vi "Finish.vi"   [LabVIEW 2015]
doc: "This VI is called just before exiting. It is expected to close I/O refnum, save collected data, etc."
uses:
  Device Refnums.ctl
  <vilib>/Rock Robotics/WPI/Utilities/WPI_GetSetVariantRefNum.vi
  ADIS16448-RoboRIO-Driver/trunk/LabVIEW/ADI MXP IMU/FRC ADI MXP IMU.lvlib
types:
  T1 = typedef "Device Refnums.ctl" = string
  T2 = typedef "WPI_JoystickDevRef.ctl" = cluster{"Device":T3}
  T3 = typedef "WPI_JoystickDeviceEnum.ctl" = enum16{"USB 0", "USB 1", "USB 2", "USB 3", "USB 4", "USB 5"}
  T4 = typedef "WPI_RobotDriveDevRef.ctl" = cluster{"DevStatus":errorcluster, "Motors[]":T5[], "Square Inputs":bool, "Max Output":dbl}
  T5 = typedef "WPI_MotorControlDeviceRef.ctl" = cluster{"DeviceStatus":errorcluster, "Type":T6, "PWM":cluster{"PWM Channel":T7, "DeadBand":T8}, "CAN":cluster{"Device Number":u8, "Control Mode":T9, "Semaphore":T10, "Max Vout":dbl, "TalonSRX Control Mode":T11}, "Invert":bool}
  T6 = typedef "WPI_MotorControlType.ctl" = enum16{"PWM", "CAN", "CANTalonSRX"}
  T7 = typedef "FPGA_DIOPWMChannel.ctl" = enum8{"PWM 0", "PWM 1", "PWM 2", "PWM 3", "PWM 4", "PWM 5", "PWM 6", "PWM 7", "PWM 8", "PWM 9", "PWM MXP 0", "PWM MXP 1", "PWM MXP 2", "PWM MXP 3", "PWM MXP 4", "PWM MXP 5", "PWM MXP 6", "PWM MXP 7", "PWM MXP 8", "PWM MXP 9", "Invalid"}
  T8 = typedef "WPI_PWMDeadband.ctl" = cluster{"Name":string, "maxPositivePwm":i32, "minPositivePwm":i32, "centerPwm":i32, "maxNegativePwm":i32, "minNegativePwm":i32, "angularRange":u16}
  T9 = typedef "WPI_CANJaguar_ControlMode.ctl" = enum8{"Percent VBus", "Current", "Speed", "Position", "Voltage"}
  T10 = typedef "Semaphore RefNum" = refnum<k1>
  T11 = typedef "WPI_CANTalonSRX_APIControlMode.ctl" = enum8{"Percent VBus", "Speed", "Position", "Slave", "Unchanged / Invalid", "Voltage Compensation", "Current", "Motion Profile"}
  T12 = typedef "WPI_EncoderDevRef.ctl" = cluster{"DevStatus":errorcluster, "EncoderIndex":T13, "CounterIndex":T14, "DistancePerCount":dbl, "Decoding Type":T15}
  T13 = typedef "FPGA_EncoderIdx.ctl" = enum8{"Enc 0", "Enc 1", "Enc 2", "Enc 3", "Enc 4", "Enc 5", "Enc 6", "Enc 7", "Invalid"}
  T14 = typedef "FPGA_CounterCtrSystemIndex.ctl" = enum8{"Ctr 0", "Ctr 1", "Ctr 2", "Ctr 3", "Ctr 4", "Ctr 5", "Ctr 6", "Ctr 7", "Invalid"}
  T15 = typedef "WPI_EncoderType.ctl" = enum16{"1x", "2x", "4x"}
  T16 = typedef "WPI_AnalogChannelDevRef.ctl" = cluster{"DevStatus":errorcluster, "Analog Channel":T17}
  T17 = typedef "FPGA_AIChannel.ctl" = enum8{"AI 0", "AI 1", "AI 2", "AI 3", "AI MXP 0", "AI MXP 1", "AI MXP 2", "AI MXP 3", "Invalid"}
  T18 = typedef "WPI_SolenoidDevRef.ctl" = cluster{"DevStatus":errorcluster, "Pneumatics Control Module":u8, "Forward Solenoid Channel":T19, "Reverse Solenoid Channel":T19}
  T19 = typedef "WPI_SolenoidChannel.ctl" = enum8{"Solenoid 0", "Solenoid 1", "Solenoid 2", "Solenoid 3", "Solenoid 4", "Solenoid 5", "Solenoid 6", "Solenoid 7", "Invalid"}
  T20 = typedef "WPI_CompressorDevRef.ctl" = cluster{"DevStatus":errorcluster, "Pneumatics Control Module":u8}
  T21 = typedef "FRC ADI MXP IMU.lvlib/WPI_AnalogDevicesIMUInterruptDevRef.ctl" = cluster{"SimpleGyroDevRef":T22, "InterruptRef":T24}
  T22 = typedef "FRC ADI MXP IMU.lvlib/WPI_AnalogDevicesIMUDevRef.ctl" = cluster{"DevStatus":errorcluster, "Handle":i32, "SPI Bus":T23, "Device Found":bool, "Sample Rate":dbl, "Device Ready":bool, "Yaw Axis":enum16{"X", "Y", "Z"}, "AHRS Algorithm":enum16{"Complementary", "Madgwick"}}
  T23 = typedef "spi_bus.ctl" = enum16{"SPI On-Board, CS0", "SPI On-Board, CS1", "SPI On-Board, CS2", "SPI On-Board, CS3", "SPI MXP", "Invalid"}
  T24 = typedef "WPI_InterruptRef.ctl" = cluster{"DevStatus":errorcluster, "InterruptIndex":T25}
  T25 = typedef "FPGA_InterruptIndex.ctl" = enum8{"0", "1", "2", "3", "4", "5", "6", "7", "Invalid"}
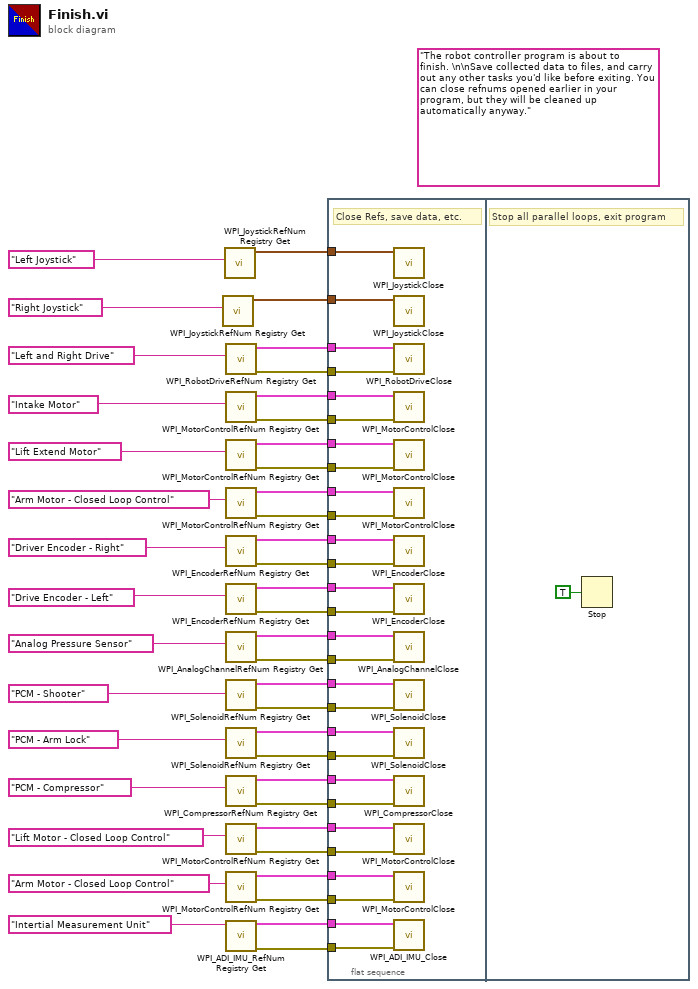
[diagram p0: block diagram]
diagram:
  (unwired) "The robot controller program is about to finish. \n\nSave collected data to files, and carry out any other tasks you'd like before exiting. You can close refnums opened earlier in your program, but they will be cleaned up automatically anyway."
  n1 = call <vilib>:"WPI_JoystickRefNum Registry Get.vi"("refnum name"=T1 "Right Joystick" ("Device Name")) -> ("JoystickDevRef"=w18:T2)  [unwired: 9 in, 1 out]
  n2 = call <vilib>:"WPI_JoystickRefNum Registry Get.vi"("refnum name"=T1 "Left Joystick" ("Device Name")) -> ("JoystickDevRef"=w17:T2)  [unwired: 9 in, 1 out]
  n3 = call <vilib>:"WPI_RobotDriveRefNum Registry Get.vi"("refnum name"=T1 "Left and Right Drive" ("Device Name")) -> ("error out"=w13:errorcluster, "RobotDriveDevRef"=w43:T4)  [unwired: 1 in, 8 out]
  n4 = call <vilib>:"WPI_MotorControlRefNum Registry Get.vi"("refnum name"=T1 "Intake Motor" ("Device Name")) -> ("error out"=w14:errorcluster, "MotorControlDevRef"=w33:T5)  [unwired: 9 in]
  n5 = call <vilib>:"WPI_MotorControlRefNum Registry Get.vi"("refnum name"=T1 "Lift Extend Motor" ("Device Name")) -> ("error out"=w12:errorcluster, "MotorControlDevRef"=w34:T5)  [unwired: 9 in]
  n6 = call <vilib>:"WPI_MotorControlRefNum Registry Get.vi"("refnum name"=T1 "Arm Motor - Closed Loop Control" ("Device Name")) -> ("error out"=w11:errorcluster, "MotorControlDevRef"=w37:T5)  [unwired: 9 in]
  n7 = call <vilib>:"WPI_EncoderRefNum Registry Get.vi"("refnum name"=T1 "Driver Encoder - Right" ("Device Name")) -> ("error out"=w10:errorcluster, "EncoderDevRef"=w35:T12)  [unwired: 9 in]
  n8 = call <vilib>:"WPI_EncoderRefNum Registry Get.vi"("refnum name"=T1 "Drive Encoder - Left" ("Device Name")) -> ("error out"=w9:errorcluster, "EncoderDevRef"=w36:T12)  [unwired: 9 in]
  n9 = call <vilib>:"WPI_AnalogChannelRefNum Registry Get.vi"("refnum name"=T1 "Analog Pressure Sensor" ("Device Name")) -> ("error out"=w4:errorcluster, "AIDeviceRef"=w42:T16)  [unwired: 9 in]
  n10 = call <vilib>:"WPI_SolenoidRefNum Registry Get.vi"("refnum name"=T1 "PCM - Shooter" ("Device Name")) -> ("error out"=w6:errorcluster, "SolenoidDevRef"=w40:T18)  [unwired: 9 in]
  n11 = call <vilib>:"WPI_SolenoidRefNum Registry Get.vi"("refnum name"=T1 "PCM - Arm Lock" ("Device Name")) -> ("error out"=w8:errorcluster, "SolenoidDevRef"=w39:T18)  [unwired: 9 in]
  n12 = call <vilib>:"WPI_CompressorRefNum Registry Get.vi"("refnum name"=T1 "PCM - Compressor" ("Device Name")) -> ("error out"=w5:errorcluster, "CompressorDevRef"=w41:T20)  [unwired: 9 in]
  n13 = call <vilib>:"WPI_MotorControlRefNum Registry Get.vi"("refnum name"=T1 "Lift Motor - Closed Loop Control" ("Device Name")) -> ("error out"=w7:errorcluster, "MotorControlDevRef"=w38:T5)  [unwired: 9 in]
  n14 = call <vilib>:"WPI_MotorControlRefNum Registry Get.vi"("refnum name"=T1 "Arm Motor - Closed Loop Control" ("Device Name")) -> ("error out"=w3:errorcluster, "MotorControlDevRef"=w2:T5)  [unwired: 9 in]
  n15 = call "WPI_ADI_IMU_RefNum Registry Get.vi"("refnum name"=T1 "Intertial Measurement Unit" ("Device Name")) -> ("error out"=w32:errorcluster, "ADI IMU Interrupt DevRef"=w31:T21)  [unwired: 9 in]
  n16 = flat-sequence {
    tunnel: w43 -> [w71]
    tunnel: w33 -> [w70]
    tunnel: w34 -> [w69]
    tunnel: w42 -> [w68]
    tunnel: w41 -> [w67]
    tunnel: w40 -> [w66]
    tunnel: w39 -> [w65]
    tunnel: w38 -> [w64]
    tunnel: w37 -> [w63]
    tunnel: w36 -> [w62]
    tunnel: w35 -> [w61]
    tunnel: w32 -> [w60]
    tunnel: w31 -> [w59]
    tunnel: w18 -> [w58]
    tunnel: w17 -> [w57]
    tunnel: w14 -> [w56]
    tunnel: w13 -> [w55]
    tunnel: w12 -> [w54]
    tunnel: w11 -> [w53]
    tunnel: w10 -> [w52]
    tunnel: w9 -> [w51]
    tunnel: w8 -> [w50]
    tunnel: w7 -> [w49]
    tunnel: w6 -> [w48]
    tunnel: w5 -> [w47]
    tunnel: w4 -> [w46]
    tunnel: w3 -> [w45]
    tunnel: w2 -> [w44]
    frame #0 {
      # "Close Refs, save data, etc."
      n17 = call <vilib>:"WPI_JoystickClose.vi"("JoystickDevRef"=w57) -> ()  [unwired: 11 in]
      n18 = call <vilib>:"WPI_JoystickClose.vi"("JoystickDevRef"=w58) -> ()  [unwired: 11 in]
      n19 = call <vilib>:"WPI_RobotDriveClose.vi"("error in (no error)"=w55, "RobotDriveDevRef"=w71) -> ()  [unwired: 10 out]
      n20 = call <vilib>:"WPI_MotorControlClose.vi"("error in (no error)"=w56, "MotorControlDevRef"=w70) -> ()  [unwired: 9 in, 1 out]
      n21 = call <vilib>:"WPI_MotorControlClose.vi"("error in (no error)"=w54, "MotorControlDevRef"=w69) -> ()  [unwired: 9 in, 1 out]
      n22 = call <vilib>:"WPI_MotorControlClose.vi"("error in (no error)"=w53, "MotorControlDevRef"=w63) -> ()  [unwired: 9 in, 1 out]
      n23 = call <vilib>:"WPI_EncoderClose.vi"("error in (no error)"=w52, "EncoderDevRef"=w61) -> ()  [unwired: 9 in, 1 out]
      n24 = call <vilib>:"WPI_EncoderClose.vi"("error in (no error)"=w51, "EncoderDevRef"=w62) -> ()  [unwired: 9 in, 1 out]
      n25 = call <vilib>:"WPI_AnalogChannelClose.vi"("error in (no error)"=w46, "AIDeviceRef"=w68) -> ()  [unwired: 9 in, 1 out]
      n26 = call <vilib>:"WPI_SolenoidClose.vi"("error in (no error)"=w48, "SolenoidDevRef"=w66) -> ()  [unwired: 9 in, 1 out]
      n27 = call <vilib>:"WPI_SolenoidClose.vi"("error in (no error)"=w50, "SolenoidDevRef"=w65) -> ()  [unwired: 9 in, 1 out]
      n28 = call <vilib>:"WPI_CompressorClose.vi"("error in (no error)"=w47, "CompressorDevRef"=w67) -> ()  [unwired: 9 in, 1 out]
      n29 = call <vilib>:"WPI_MotorControlClose.vi"("error in (no error)"=w49, "MotorControlDevRef"=w64) -> ()  [unwired: 9 in, 1 out]
      n30 = call <vilib>:"WPI_MotorControlClose.vi"("error in (no error)"=w45, "MotorControlDevRef"=w44) -> ()  [unwired: 9 in, 1 out]
      n31 = call "WPI_ADI_IMU_Close.vi"("error in"=w60, "ADI IMU Interrupt DevRef"=w59) -> ()  [unwired: 9 in, 1 out]
    }
    frame #1 {
      # "Stop all parallel loops, exit program"
      n32 = Stop(stop? (T)=TRUE ("Quit")) -> ()
    }
  }
